vi "Add test to error descriptions.vi"(4 "error descriptions in":T2, 5 "error string":string, 6 "error type":T1, 7 "pass":bool) -> (0 "error description out":T2)   [LabVIEW 2019]
uses:
  error type.ctl
  error description.ctl
  array of error description.ctl
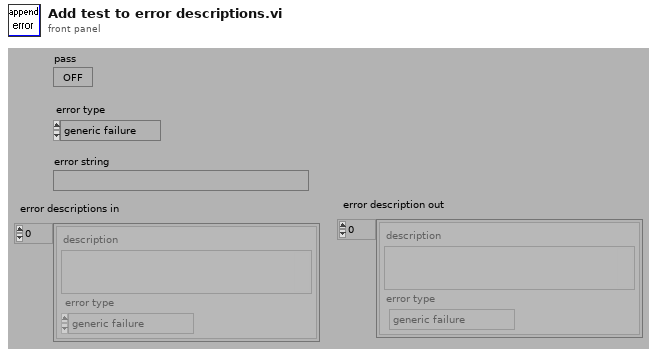
[diagram p1: front panel]
types:
  T1 = typedef "error type.ctl" = enum32{"generic failure", "boundary case", "precision", "expected error"}
  T2 = typedef "array of error description.ctl" = T3[]
  T3 = typedef "error description.ctl" = cluster{"description":string, "error type":T1}
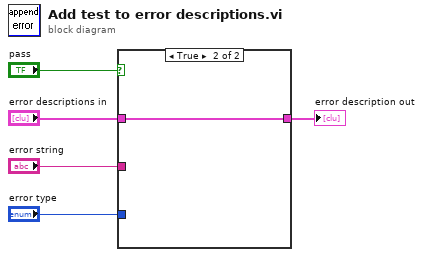
[diagram p0: block diagram]
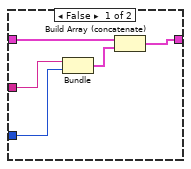
[diagram p2: hidden frame]
diagram:
  n1 = case shown="True" "pass" {
    tunnel: "error descriptions in" -> [w10 w11]
    tunnel: [w9 w11] -> w4
    tunnel: "error string" -> [w7 _]
    tunnel: "error type" -> [w6 _]
    frame False {
      n2 = Bundle("error string"=w7, "error type"=w6) -> (w8:cluster{"error string":string, "error type":T1})  [unwired: 1 in]
      n3 = Build Array (concatenate)(w10, w8) -> (w9:T2)
    }
    frame True {
    }
  }
  "error description out" <- w4
